vi "Dispose.vi"(0 "object in":refnum<class "TowerLight.lvclass">, 5 "error in (no error)":errorcluster) -> (14 "object out":refnum<class "TowerLight.lvclass">, 19 "error out":errorcluster)   [LabVIEW 2014, in "TowerLight.lvclass"]
uses:
  TowerLight.lvclass
  TowerLight.lvclass/TowerLight.ctl
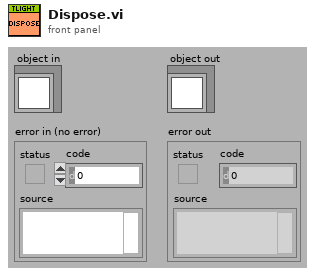
[diagram p1: front panel]
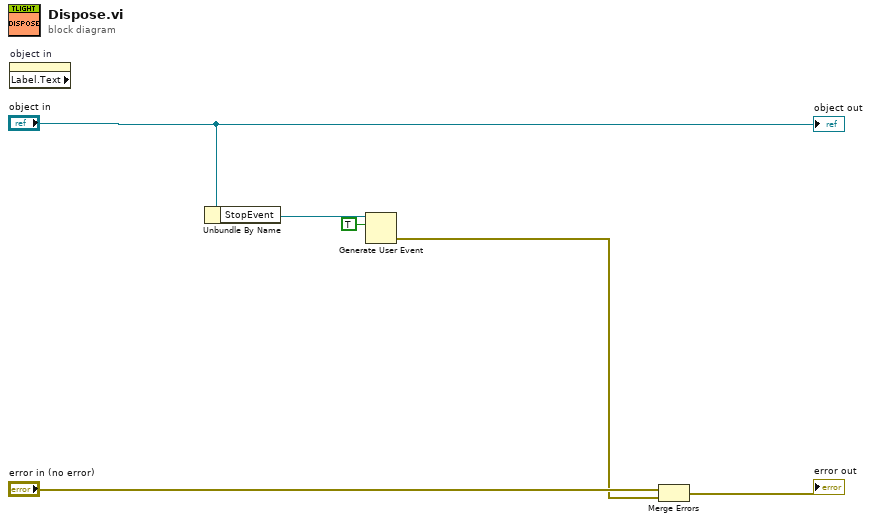
[diagram p0: block diagram]
diagram:
  n1 = property on="object in" class="LVClassControl (strict)" props=["Label", "Text"]() -> ()  [unwired: 2 in, 3 out]
  n2 = Unbundle By Name("object in") -> ("StopEvent"=w4:refnum<user-event>)
  n3 = Generate User Event(user event=w4, event data cluster=TRUE ("event data")) -> (error out=w1:errorcluster)  [unwired: 2 in, 1 out]
  n4 = Merge Errors("error in (no error)", w1) -> (→"error out":errorcluster)
  "object out" <- "object in"
